vi "Write.vi"(8 "error in (no error)":errorcluster, 10 "Write Buffer":string, 11 "VISA resource name":refnum<visa-resource-name>) -> (0 "error out":errorcluster, 2 "Return Count":u32, 3 "VISA resource name out":refnum<visa-resource-name>)   [LabVIEW 2013, in "LeCroy Wave Series.lvlib"]
doc: "Writes data from write buffer to the device or interface specified by VISA resource name. It is modified for beater device communication over TCP/IP.\n\n<B>Note:</B>\n\nThis is a low-level Write VI that can be used to send commands to the instrument for functionality not supported by the driver."
uses:
  LeCroy Wave Series.lvlib
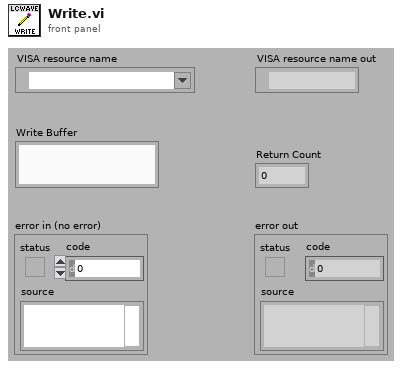
[diagram p1: front panel]
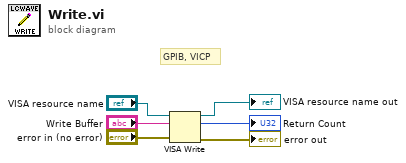
[diagram p0: block diagram]
diagram:
  # "GPIB, VICP"
  n1 = VISA Write(VISA resource name="VISA resource name", write buffer="Write Buffer", error in (no error)="error in (no error)") -> (VISA resource name out=→"VISA resource name out":refnum<visa-resource-name>, return count=→"Return Count":u32, error out=→"error out":errorcluster)
